vi "Assymetric_Sine_Wave.vi"(9 "Ts":dbl=1.0, 10 "Ub":dbl=1.0, 11 "samples":i32=128) -> (1 "offset":dbl, 2 "amplitude":dbl, 3 "Assymetric Sign Wave":dbl[](array[numeric]))   [LabVIEW 2011]
uses:
  <vilib>/Analysis/baseanly.llb/Scale 1D.vi
  <vilib>/Analysis/NI_AALBase.lvlib
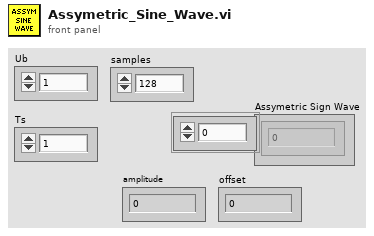
[diagram p1: front panel]
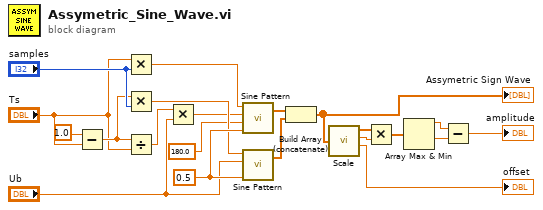
[diagram p0: block diagram]
diagram:
  w21 = 0.5 ("cycles")
  n1 = Subtract(x=1.0, y="Ts") -> (x-y=w10:dbl)
  n2 = Multiply(x="Ts", y="samples") -> (x*y=w20:dbl)
  n3 = Multiply(x=w10, y="samples") -> (x*y=w17:dbl)
  n4 = Divide(x=w10, y="Ts") -> (x/y=w11:dbl)
  n5 = Multiply(x=w11, y="Ub") -> (x*y=w15:dbl)
  n6 = call <vilib>:"Sine Pattern.vi"("cycles"=w21, "phase(degrees)"=180.0, "amplitude"=w15, "samples"=w20) -> ("Sinusoidal Pattern"=w14:dbl[])  [unwired: 1 out]
  n7 = call <vilib>:"Sine Pattern.vi"("cycles"=w21, "amplitude"="Ub", "samples"=w17) -> ("Sinusoidal Pattern"=w13:dbl[])  [unwired: 1 in, 1 out]
  n8 = Build Array (concatenate)(w14, w13) -> (w8:dbl[])
  "Assymetric Sign Wave" <- w8
  n9 = call-poly <vilib>:"Scale.vi"("X"=w8) -> ("Y=(X-offset)/scale"=w6:dbl[], "scale"=w7:dbl, "offset"=→"offset":dbl)  [unwired: 1 out]
  n10 = Multiply(x=w6, y=w7) -> (x*y=w5:dbl[])
  n11 = Array Max & Min(array=w5) -> (max value=w4:dbl, min value=w3:dbl)  [unwired: 2 out]
  n12 = Subtract(x=w4, y=w3) -> (x-y=→"amplitude":dbl)
